vi "util_tokenize_string.vi"(8 "error in (no error)":errorcluster, 10 "delimiter":string, 11 "input_string":string) -> (0 "error out":errorcluster, 2 "match []":string[](array[string]), 3 "before_match []":string[](array[string]))   [LabVIEW 2015, in "lv-bin.lvlib" / "v1.lvlib"]
uses:
  v1.lvlib
  <vilib>/regexp/Match Regular Expression.xnode
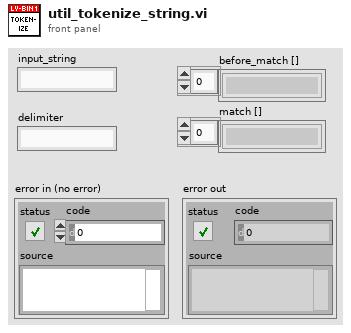
[diagram p1: front panel]
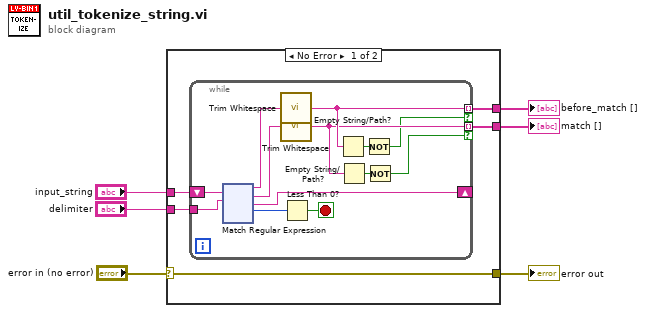
[diagram p0: block diagram]
diagram:
  n1 = case shown="No Error" "error in (no error)" {
    selector: "error in (no error)" -> [w11 w139]
    tunnel: "delimiter" -> [w9 _]
    tunnel: [w8 _] -> w5
    tunnel: "input_string" -> [w10 _]
    tunnel: [w11 w139] -> w2
    tunnel: [w7 _] -> w1
    frame No Error {
      n2 = while {
        shift-right: [w24] -> _
        shift-left: w10 -> [w20]
        tunnel: [w15] -> w8 mode=indexing if=w13
        tunnel: w9 -> [w22]
        tunnel: [w14] -> w7 mode=indexing if=w12
        stop <- w23 stop-if-true
        n3 = xnode "Match Regular Expression"("input string"=w20, "regular expression"=w22) -> ("before match"=w21:string, "whole match"=w18:string, "after match"=w24:string, "offset past match"=w19:i32)  [unwired: 4 in, 1 out]
        n4 = call <vilib>:"Trim Whitespace.vi"("string"=w21) -> ("trimmed string"=w15:string)  [unwired: 1 in]
        n5 = call <vilib>:"Trim Whitespace.vi"("string"=w18) -> ("trimmed string"=w14:string)  [unwired: 1 in]
        n6 = Less Than 0?(x=w19) -> (x < 0?=w23:bool)
        n7 = Empty String/Path?(string/path=w15) -> (empty?=w17:bool)
        n8 = Empty String/Path?(string/path=w14) -> (empty?=w16:bool)
        n9 = Not(x=w17) -> (.not. x?=w13:bool)
        n10 = Not(x=w16) -> (.not. x?=w12:bool)
      }
    }
    frame Error {
    }
  }
  "before_match []" <- w5
  "error out" <- w2
  "match []" <- w1
